vi "ContactsAC.vi"() -> ()   [LabVIEW 2015]
uses:
  <vilib>/Utility/file.llb/Write To Spreadsheet File (DBL).vi
panel:
  out "2 probe R":dbl
  out "Array":bool[][](array[boolean])
  in  "Resistor":u16(ring) items=["10 MOhm", "1 MOhm", "100 kOhm", "10 kOhm", "1 kOhm"]
  in  "GPIB Address":string="1"
  in  "Record new values":bool
  out "Y (V)":dbl
  out "X (V)":dbl
  out "Harmonic #":dbl
  out "Phase":dbl
  out "Oscillator (V)":dbl
  out "Frequency (Hz)":dbl
  out "Time Constant":u16(ring) items=["10 us", "30 us", "100 us", "300 us", "1 ms", "3 ms", "10 ms", "30 ms", "100 ms", "300 ms", "1 s", "3 s", "10 s", "30 s", "100 s", "300 s", "1 ks", "3 ks", "10 ks", "30 ks"]
  out "Sensitivity":u16(ring) items=["2 nV", "5 nV", "10 nV", "20 nV", "50 nV", "100 nV", "200 nV", "500 nV", "1 uV", "2 uV", "5 uV", "10 uV", "20 uV", "50 uV", "100 uV", "200 uV", "500 uV", "1 mV", "2 mV", "5 mV", "10 mV", "20 mV", "50 mV", "100 mV", "200 mV", "500 mV", "1 V"]
  in  "ON/OFF channel":bool
  in  "error in (no error)":errorcluster
  out "error out":errorcluster
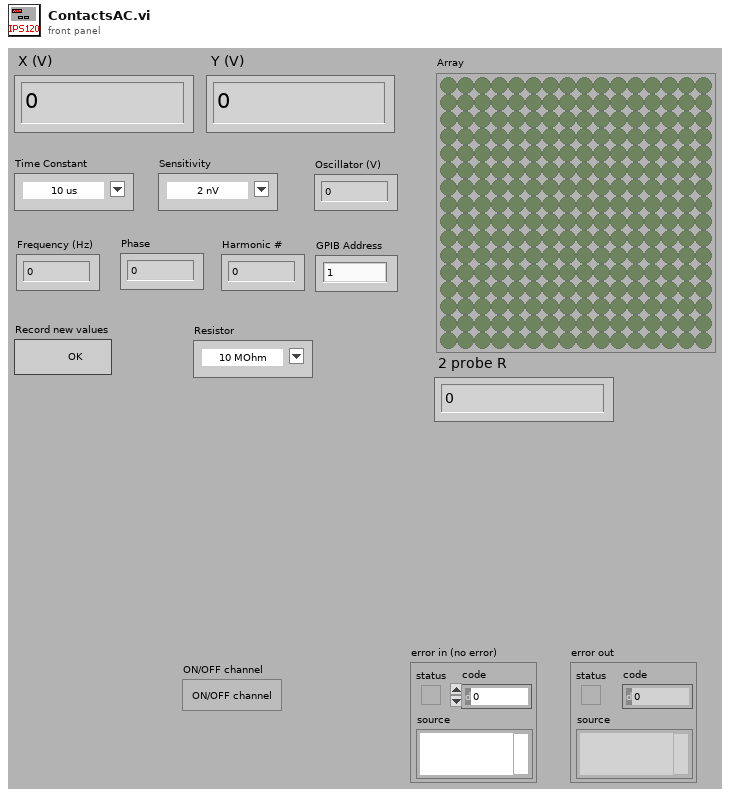
[diagram p1: front panel]
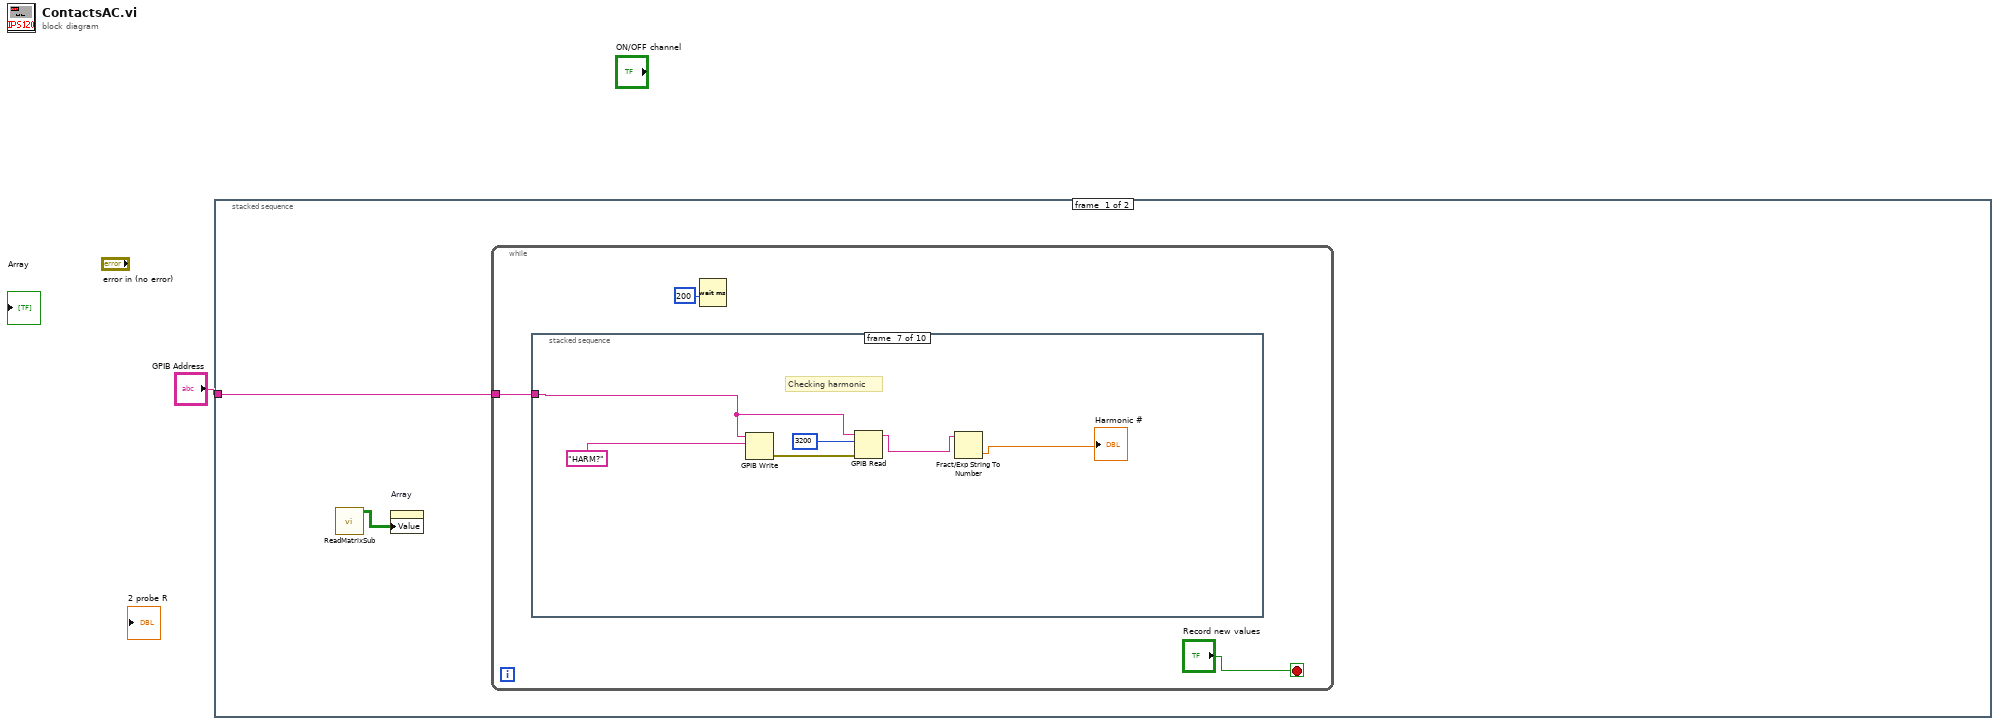
[diagram p0: block diagram]
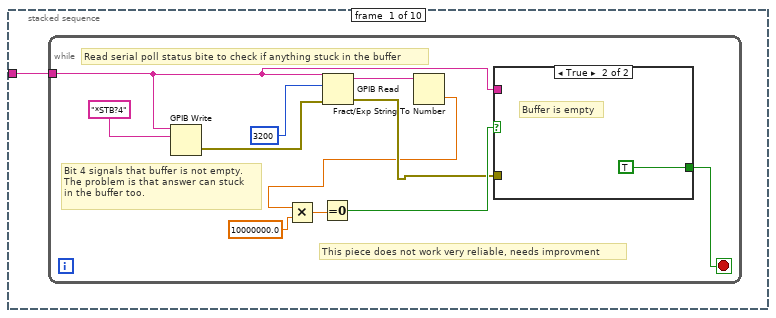
[diagram p2: hidden frame]
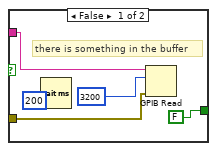
[diagram p3: hidden frame]
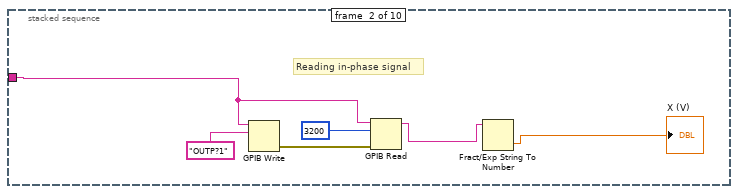
[diagram p4: hidden frame]
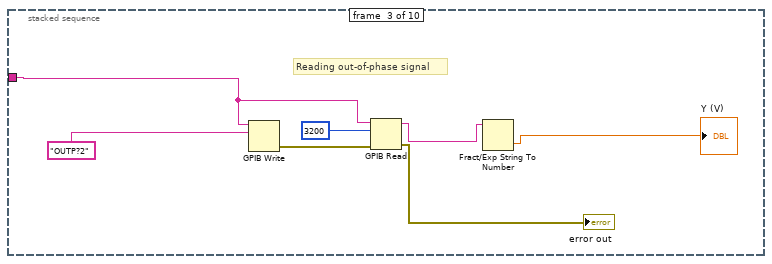
[diagram p5: hidden frame]
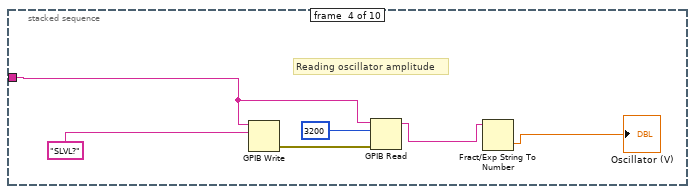
[diagram p6: hidden frame]
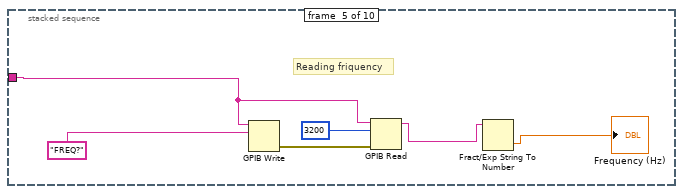
[diagram p7: hidden frame]
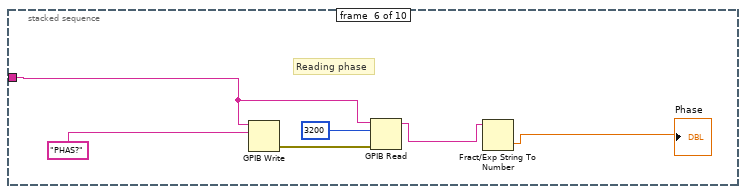
[diagram p8: hidden frame]
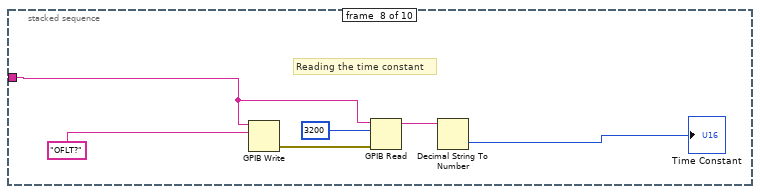
[diagram p9: hidden frame]
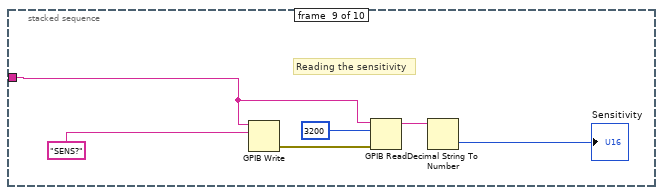
[diagram p10: hidden frame]
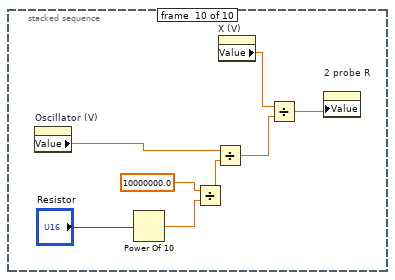
[diagram p11: hidden frame]
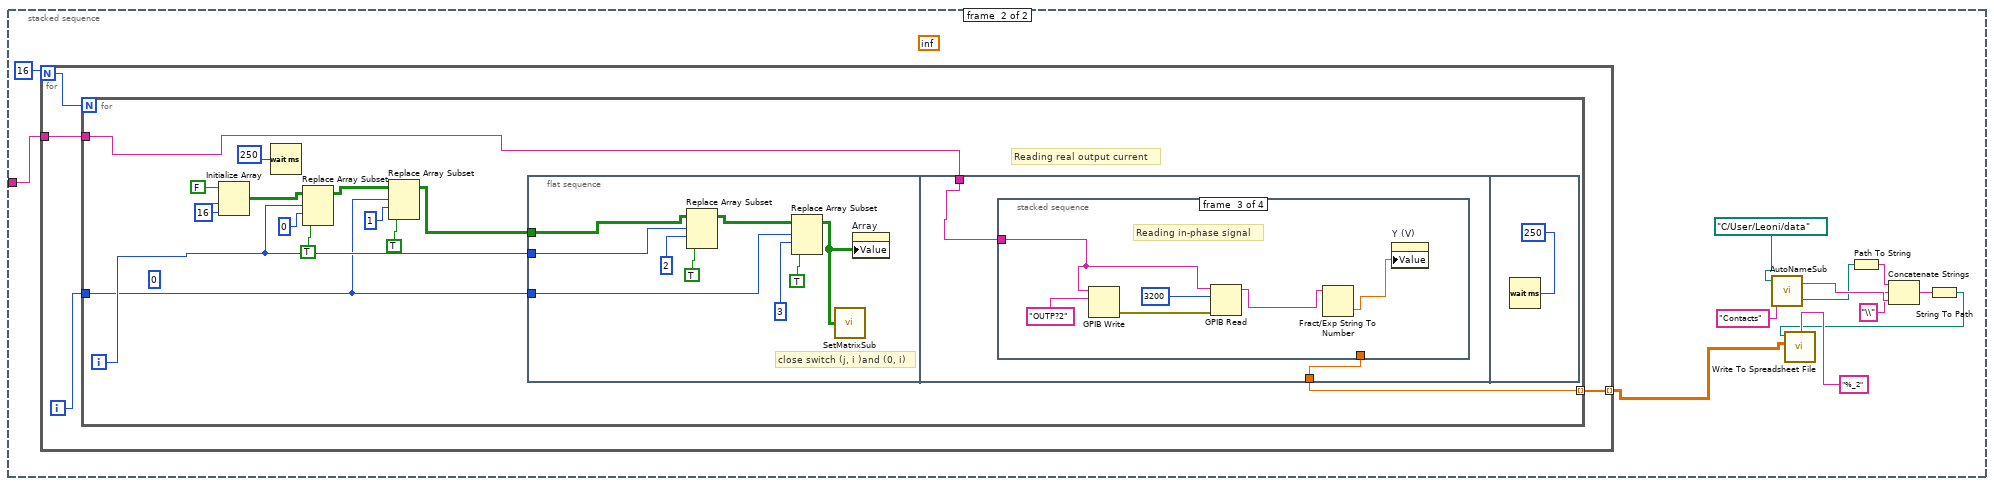
[diagram p12: hidden frame]
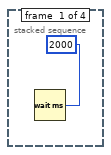
[diagram p13: hidden frame]
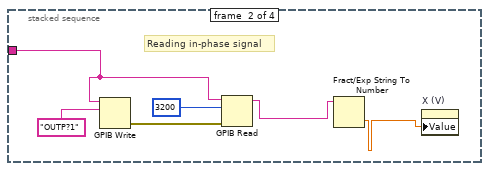
[diagram p14: hidden frame]
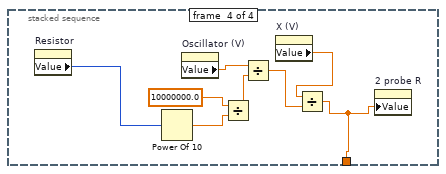
[diagram p15: hidden frame]
diagram:
  n1 = stacked-sequence {
    tunnel: "GPIB Address" -> [w3 w92]
    frame #0 {
      n2 = call "ReadMatrixSub.vi"() -> ("Array"=w2:bool[][])  [unwired: 9 in, 2 out]
      n3 = property on="Array" class="Arr (strict)"("Value"=w2) -> ()  [unwired: 2 in, 2 out]
      n4 = while {
        tunnel: w3 -> [w6]
        stop <- "Record new values" stop-if-true
        n5 = stacked-sequence {
          tunnel: w6 -> [w7 w25 w32 w38 w44 w50 w56 w62 w68 _]
          frame #0 {
            n6 = while {
              tunnel: w7 -> [w14]
              stop <- w13 stop-if-true
              # "Bit 4 signals that buffer is not empty.\nThe problem is that answer can stuck\nin the buffer too."
              # "Read serial poll status bite to check if anything stuck in the buffer"
              # "This piece does not work very reliable, needs improvment"
              n7 = GPIB Write(0:w14, 1:"*STB?4") -> (6:w17:errorcluster)  [unwired: 3 in, 1 out]
              n8 = GPIB Read(0:w14, 1:3200, 3:w17) -> (5:w15:string, 7:w11:errorcluster)  [unwired: 2 in, 1 out]
              n9 = Fract/Exp String To Number(string=w15) -> (number=w9:dbl)  [unwired: 3 in, 1 out]
              n10 = Multiply(x=w9, y=10000000.0) -> (x*y=w10:dbl)
              n11 = Equal To 0?(x=w10) -> (x = 0?=w12:bool)
              n12 = case shown="True" w12 {
                tunnel: w14 -> [w22 _]
                tunnel: [FALSE TRUE] -> w13
                tunnel: w11 -> [w20 _]
                frame False {
                  # "there is something in the buffer"
                  n13 = Wait (ms)(milliseconds to wait=200) -> ()  [unwired: 1 out]
                  n14 = GPIB Read(0:w22, 1:3200, 3:w20) -> ()  [unwired: 2 in, 3 out]
                }
                frame True {
                  # "Buffer is empty"
                }
              }
            }
          }
          frame #1 {
            # "Reading in-phase signal"
            n15 = GPIB Write(0:w25, 1:"OUTP?1") -> (6:w30:errorcluster)  [unwired: 3 in, 1 out]
            n16 = GPIB Read(0:w25, 1:3200, 3:w30) -> (5:w27:string)  [unwired: 2 in, 2 out]
            n17 = Fract/Exp String To Number(string=w27) -> (number=→"X (V)":dbl)  [unwired: 3 in, 1 out]
          }
          frame #2 {
            # "Reading out-of-phase signal"
            n18 = GPIB Write(0:w32, 1:"OUTP?2") -> (6:w37:errorcluster)  [unwired: 3 in, 1 out]
            n19 = GPIB Read(0:w32, 1:3200, 3:w37) -> (5:w34:string, 7:→"error out":errorcluster)  [unwired: 2 in, 1 out]
            n20 = Fract/Exp String To Number(string=w34) -> (number=→"Y (V)":dbl)  [unwired: 3 in, 1 out]
          }
          frame #3 {
            # "Reading oscillator amplitude"
            n21 = GPIB Write(0:w38, 1:"SLVL?") -> (6:w43:errorcluster)  [unwired: 3 in, 1 out]
            n22 = GPIB Read(0:w38, 1:3200, 3:w43) -> (5:w40:string)  [unwired: 2 in, 2 out]
            n23 = Fract/Exp String To Number(string=w40) -> (number=→"Oscillator (V)":dbl)  [unwired: 3 in, 1 out]
          }
          frame #4 {
            # "Reading friquency"
            n24 = GPIB Write(0:w44, 1:"FREQ?") -> (6:w49:errorcluster)  [unwired: 3 in, 1 out]
            n25 = GPIB Read(0:w44, 1:3200, 3:w49) -> (5:w46:string)  [unwired: 2 in, 2 out]
            n26 = Fract/Exp String To Number(string=w46) -> (number=→"Frequency (Hz)":dbl)  [unwired: 3 in, 1 out]
          }
          frame #5 {
            # "Reading phase"
            n27 = GPIB Write(0:w50, 1:"PHAS?") -> (6:w55:errorcluster)  [unwired: 3 in, 1 out]
            n28 = GPIB Read(0:w50, 1:3200, 3:w55) -> (5:w52:string)  [unwired: 2 in, 2 out]
            n29 = Fract/Exp String To Number(string=w52) -> (number=→"Phase":dbl)  [unwired: 3 in, 1 out]
          }
          frame #6 {
            # "Checking harmonic"
            n30 = GPIB Write(0:w56, 1:"HARM?") -> (6:w61:errorcluster)  [unwired: 3 in, 1 out]
            n31 = GPIB Read(0:w56, 1:3200, 3:w61) -> (5:w58:string)  [unwired: 2 in, 2 out]
            n32 = Fract/Exp String To Number(string=w58) -> (number=→"Harmonic #":dbl)  [unwired: 3 in, 1 out]
          }
          frame #7 {
            # "Reading the time constant"
            n33 = GPIB Write(0:w62, 1:"OFLT?") -> (6:w67:errorcluster)  [unwired: 3 in, 1 out]
            n34 = GPIB Read(0:w62, 1:3200, 3:w67) -> (5:w64:string)  [unwired: 2 in, 2 out]
            n35 = Decimal String To Number(string=w64) -> (number=→"Time Constant":i32)  [unwired: 2 in, 1 out]
          }
          frame #8 {
            # "Reading the sensitivity"
            n36 = GPIB Write(0:w68, 1:"SENS?") -> (6:w73:errorcluster)  [unwired: 3 in, 1 out]
            n37 = GPIB Read(0:w68, 1:3200, 3:w73) -> (5:w70:string)  [unwired: 2 in, 2 out]
            n38 = Decimal String To Number(string=w70) -> (number=→"Sensitivity":i32)  [unwired: 2 in, 1 out]
          }
          frame #9 {
            n39 = property on="Oscillator (V)" class="DigNum (strict)"() -> ("Value"=w77:dbl)  [unwired: 2 in, 2 out]
            n40 = Power Of 10(x="Resistor") -> (10^x=w79:dbl)
            n41 = Divide(x=10000000.0, y=w79) -> (x/y=w78:dbl)
            n42 = Divide(x=w77, y=w78) -> (x/y=w75:dbl)
            n43 = property on="X (V)" class="DigNum (strict)"() -> ("Value"=w76:dbl)  [unwired: 2 in, 2 out]
            n44 = Divide(x=w76, y=w75) -> (x/y=w74:dbl)
            n45 = property on="2 probe R" class="DigNum (strict)"("Value"=w74) -> ()  [unwired: 2 in, 2 out]
          }
        }
        n46 = Wait (ms)(milliseconds to wait=200) -> ()  [unwired: 1 out]
      }
    }
    frame #1 {
      (unwired) inf
      n47 = for {
        N: 16 -> [w96]
        tunnel: w92 -> [w95]
        tunnel: [w94] -> w82 mode=indexing
        i -> [w97]
        n48 = for {
          N: w96 -> [_]
          tunnel: w97 -> [w98]
          tunnel: w95 -> [w110]
          tunnel: [w109] -> w94 mode=indexing
          i -> [w111]
          w107 = 16
          (unwired) 0
          # "Reading real output current"
          n49 = Initialize Array(FALSE, w107, w107) -> (w106:bool[][])
          n50 = Wait (ms)(milliseconds to wait=250) -> ()  [unwired: 1 out]
          n51 = Replace Array Subset(array=w106, new element=TRUE, index (row)=w111, index (col)=0) -> (w101:bool[][])
          n52 = Replace Array Subset(array=w101, new element=TRUE, index (row)=w98, index (col)=1) -> (w99:bool[][])
          n53 = flat-sequence {
            tunnel: w99 -> [w117]
            tunnel: w98 -> [w114]
            tunnel: w111 -> [w116]
            tunnel: w110 -> [w122]
            tunnel: [w121] -> w109
            frame #0 {
              # "close switch (j, i )and (0, i)"
              n54 = Replace Array Subset(array=w117, new element=TRUE, index (row)=w116, index (col)=2) -> (w118:bool[][])
              n55 = Replace Array Subset(array=w118, new element=TRUE, index (row)=w114, index (col)=3) -> (w112:bool[][])
              n56 = call "SetMatrixSub.vi"("Array"=w112) -> ()  [unwired: 1 in]
              n57 = property on="Array" class="Arr (strict)"("Value"=w112) -> ()  [unwired: 2 in, 2 out]
            }
            frame #1 {
              n58 = stacked-sequence {
                tunnel: w122 -> [_ w125 w131 _]
                tunnel: [_ _ _ w136] -> w121
                frame #0 {
                  n59 = Wait (ms)(milliseconds to wait=2000) -> ()  [unwired: 1 out]
                }
                frame #1 {
                  # "Reading in-phase signal"
                  n60 = GPIB Write(0:w125, 1:"OUTP?1") -> (6:w129:errorcluster)  [unwired: 3 in, 1 out]
                  n61 = GPIB Read(0:w125, 1:3200, 3:w129) -> (5:w126:string)  [unwired: 2 in, 2 out]
                  n62 = Fract/Exp String To Number(string=w126) -> (number=w124:dbl)  [unwired: 3 in, 1 out]
                  n63 = property on="X (V)" class="DigNum (strict)"("Value"=w124) -> ()  [unwired: 2 in, 2 out]
                }
                frame #2 {
                  # "Reading in-phase signal"
                  n64 = GPIB Write(0:w131, 1:"OUTP?2") -> (6:w135:errorcluster)  [unwired: 3 in, 1 out]
                  n65 = GPIB Read(0:w131, 1:3200, 3:w135) -> (5:w132:string)  [unwired: 2 in, 2 out]
                  n66 = Fract/Exp String To Number(string=w132) -> (number=w130:dbl)  [unwired: 3 in, 1 out]
                  n67 = property on="Y (V)" class="DigNum (strict)"("Value"=w130) -> ()  [unwired: 2 in, 2 out]
                }
                frame #3 {
                  n68 = property on="Resistor" class="Ring (strict)"() -> ("Value"=w137:u16)  [unwired: 2 in, 2 out]
                  n69 = Power Of 10(x=w137) -> (10^x=w142:dbl)
                  n70 = property on="Oscillator (V)" class="DigNum (strict)"() -> ("Value"=w138:dbl)  [unwired: 2 in, 2 out]
                  n71 = Divide(x=10000000.0, y=w142) -> (x/y=w141:dbl)
                  n72 = Divide(x=w138, y=w141) -> (x/y=w140:dbl)
                  n73 = property on="X (V)" class="DigNum (strict)"() -> ("Value"=w139:dbl)  [unwired: 2 in, 2 out]
                  n74 = Divide(x=w139, y=w140) -> (x/y=w136:dbl)
                  n75 = property on="2 probe R" class="DigNum (strict)"("Value"=w136) -> ()  [unwired: 2 in, 2 out]
                }
              }
            }
            frame #2 {
              n76 = Wait (ms)(milliseconds to wait=250) -> ()  [unwired: 1 out]
            }
          }
        }
      }
      n77 = call "AutoNameSub.vi"("Custom Folder"="Contacts", "User Data Folder"=path "C:/User/Leoni/data") -> ("created path"=w87:path, "String"=w88:string)  [unwired: 2 in]
      n78 = Path To String(path=w87) -> (string=w86:string)
      n79 = Concatenate Strings(w86, "\\", w88) -> (w84:string)
      n80 = String To Path(string=w84) -> (path=w89:path)
      n81 = call-poly <vilib>:"Write To Spreadsheet File.vi"("format (%.3f)"="%_2", "2D data"=w82, "file path (dialog if empty)"=w89) -> ()  [unwired: 5 in, 1 out]
    }
  }
